vi "reference_signal.vi"(8 "error in (no error)":errorcluster, 9 "Phase (degrees)":dbl, 10 "sampling info":cluster{"Fs":dbl, "#s":dbl}={"Fs"=200000.0, "#s"=100000.0} {"Fs" format="%.2p"}, 11 "frequency":dbl) -> (0 "error out":errorcluster, 2 "ref 90":waveform(dbl), 3 "ref":waveform(dbl))   [LabVIEW 2015]
uses:
  <vilib>/Analysis/2dsp.llb/Real FFT.vi
  <vilib>/Analysis/2dsp.llb/Inverse Real FFT.vi
  lock-in reference global.vi
  <vilib>/measure/NI_MABase.lvlib
  <vilib>/Analysis/NI_AALPro.lvlib
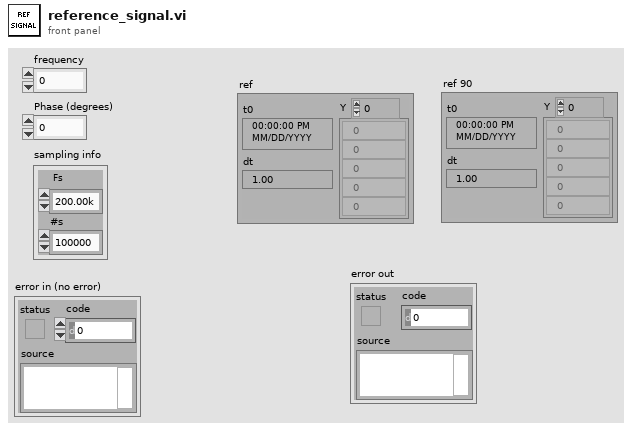
[diagram p1: front panel]
types:
  T1 = enum16{"Sine Wave", "Triangle Wave", "Square Wave", "Sawtooth Wave"}
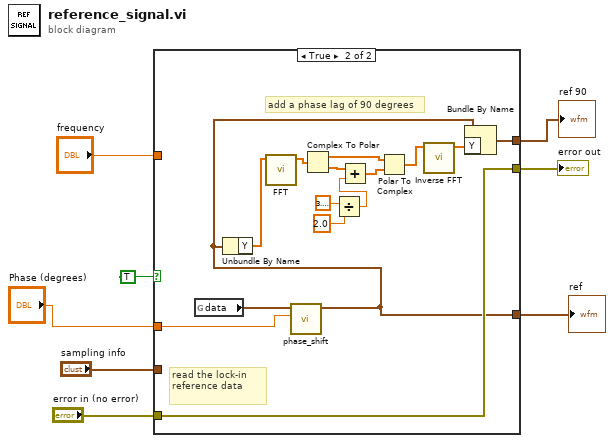
[diagram p0: block diagram]
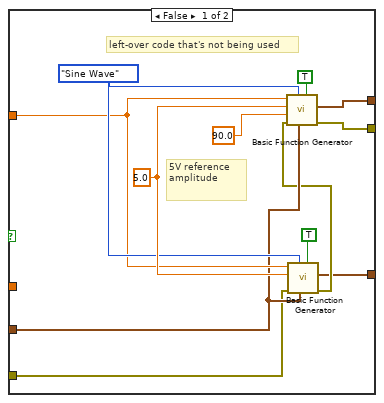
[diagram p2: hidden frame]
diagram:
  n1 = case shown="True" TRUE {
    tunnel: "frequency" -> [w15 _]
    tunnel: "sampling info" -> [w14 _]
    tunnel: "error in (no error)" -> [w13 w24]
    tunnel: [w11 w24] -> w5
    tunnel: [w10 w25] -> w4
    tunnel: [w9 w23] -> w3
    tunnel: "Phase (degrees)" -> [_ w21]
    frame False {
      w17 = T1."Sine Wave" ("signal type")
      w18 = 5.0 ("amplitude")
      # "left-over code that's not being used"
      # "5V reference amplitude"
      n2 = call <vilib>:"Basic Function Generator.vi"("reset signal"=TRUE, "sampling info"=w14, "signal type"=w17, "error in (no error)"=w13, "amplitude"=w18, "frequency"=w15) -> ("error out"=w12:errorcluster, "signal out"=w9:waveform(dbl))  [unwired: 3 in, 1 out]
      n3 = call <vilib>:"Basic Function Generator.vi"("reset signal"=TRUE, "sampling info"=w14, "signal type"=w17, "error in (no error)"=w12, "phase"=90.0 ("y"), "amplitude"=w18, "frequency"=w15) -> ("error out"=w11:errorcluster, "signal out"=w10:waveform(dbl))  [unwired: 2 in, 1 out]
    }
    frame True {
      # "add a phase lag of 90 degrees"
      # "read the lock-in reference data"
      n4 = global read "lock-in reference global.vi" "data"() -> (w22:waveform(dbl))
      n5 = call "phase_shift.vi"("Phase (degrees)"=w21, "waveform"=w22) -> ("output waveform"=w23:waveform(dbl))  [unwired: 9 in]
      n6 = Unbundle By Name(w23) -> ("Y"=w35:dbl[])
      n7 = call-poly <vilib>:"FFT.vi"("X"=w35) -> ("FFT {X}"=w34:cdb[])  [unwired: 9 in, 1 out]
      n8 = Complex To Polar(r * e^(i*theta)=w34) -> (r=w32:dbl[], theta=w33:dbl[])
      n9 = Divide(x=3.141592653589793, y=2.0) -> (x/y=w26:dbl)
      n10 = Add(x=w33, y=w26) -> (x+y=w30:dbl[])
      n11 = Polar To Complex(1:w30, 2:w32) -> (0:w31:cdb[])
      n12 = call-poly <vilib>:"Inverse FFT.vi"("FFT {X}"=w31) -> ("X"=w29:dbl[])  [unwired: 9 in, 1 out]
      n13 = Bundle By Name(cluster=w23, "Y"=w29) -> (w25:waveform(dbl))
    }
  }
  "error out" <- w5
  "ref 90" <- w4
  "ref" <- w3
